vi "gfitsio-read-column-datetime.vi"(7 "column":string, 8 "error in (no error)":errorcluster, 9 "row":i32, 11 "gfits refnum":T1) -> (0 "error out":errorcluster, 2 "data":timestamp, 3 "dup gfits refnum":T1)   [LabVIEW 2024, in "gfitsio.lvlib"]
doc: "Read elements from an ASCII or binary table column."
uses:
  gfitsio.lvlib
  gfitsio-refnum.ctl
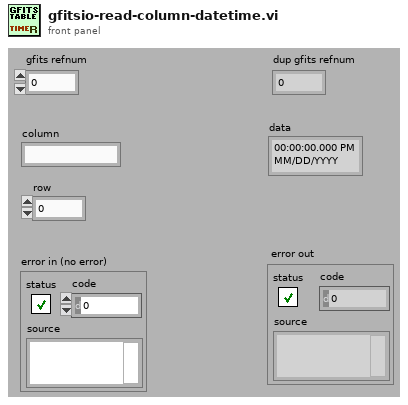
[diagram p1: front panel]
types:
  T1 = typedef "gfitsio.lvlib/gfitsio-refnum.ctl" = u64
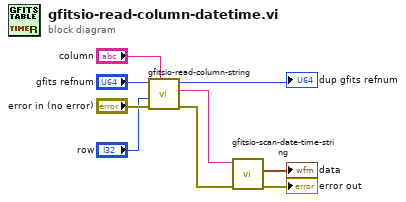
[diagram p0: block diagram]
diagram:
  n1 = call "gfitsio-read-column-string.vi"("column"="column", "error in (no error)"="error in (no error)", "row"="row", "gfits refnum"="gfits refnum") -> ("error out"=w9:errorcluster, "data"=w8:string, "dup gfits refnum"=→"dup gfits refnum":T1)  [unwired: 5 in]
  n2 = call "gfitsio-scan-date-time-string.vi"("error in (no error)"=w9, "date/time string"=w8) -> ("error out"=→"error out":errorcluster, "timestamp"=→"data":timestamp)  [unwired: 8 out]
